vi "Hardware - Buffered Counter Time.vi"(7 "Counter Time Function (Read Timer)":T1=enum."Read Timer", 8 "error in (no error)":errorcluster, 11 "Counter Task In":refnum<k21>) -> (0 "error out":errorcluster, 3 "Timer Value (ms)":dbl caption="Time Value (ms)" format="%#.6g")   [LabVIEW 2010, in "Core SubVIs.lvlib"]
uses:
  Core SubVIs.lvlib
  Controls/TYPE - Count Time Method.ctl
  <vilib>/DAQmx/read.llb/DAQmx Read (Counter 1D U32 1Chan NSamp).vi
  <vilib>/daqmx/miscellaneous.llb/DAQmx Fill In Error Info.vi
  Program Files/National Instruments/LabVIEW 2010/resource/objmgr/daqmx.rc
panel:
  in  "Timebase Rate (10 MHz Default)":dbl=10000000.0 format="%#_6p"
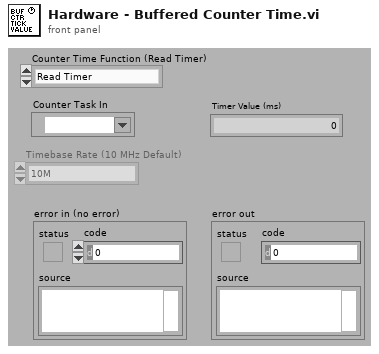
[diagram p1: front panel]
types:
  T1 = typedef "Core SubVIs.lvlib/TYPE - Count Time Method.ctl" = enum16{"Start Timer Task", "Read Timer", "Reset Timer", "Clear Timer Task"}
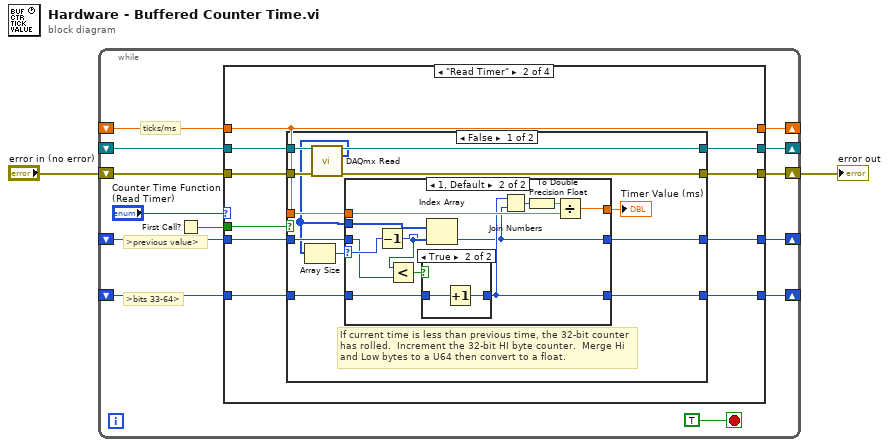
[diagram p0: block diagram]
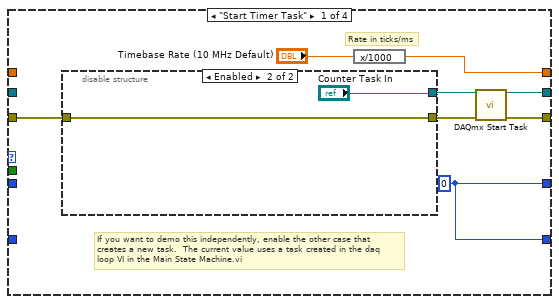
[diagram p2: hidden frame]
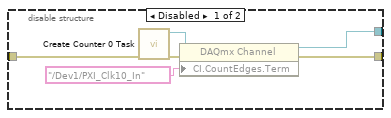
[diagram p3: hidden frame]
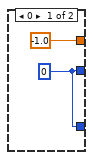
[diagram p4: hidden frame]
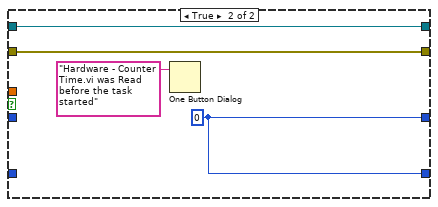
[diagram p6: hidden frame]
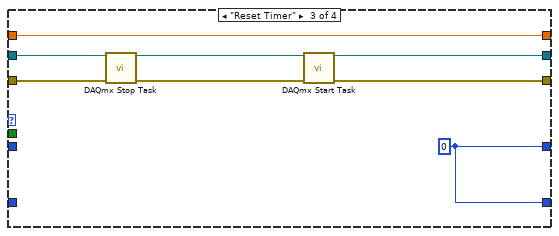
[diagram p7: hidden frame]
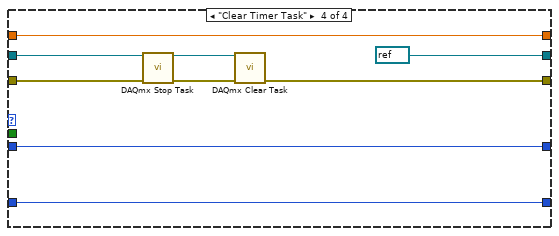
[diagram p8: hidden frame]
diagram:
  n1 = while {
    shift-right: [w12] -> _
    shift-left: _ -> [w15]
    shift-right: [w11] -> w1
    shift-left: "error in (no error)" -> [w14]
    shift-right: [w9] -> _
    shift-left: _ -> [w8]
    shift-right: [w5] -> _
    shift-left: _ -> [w6]
    shift-right: [w3] -> _
    shift-left: _ -> [w4]
    stop <- TRUE stop-if-true
    # ">bits 33-64>"
    # ">previous value>"
    # "ticks/ms"
    n2 = First Call?() -> (First Call?: T/F=w7:bool)
    n3 = case shown="\"Read Timer\"" "Counter Time Function (Read Timer)" {
      tunnel: w15 -> [_ w41 w82 w89]
      tunnel: w14 -> [w20 w40 w81 w88]
      tunnel: [w17 w39 w78 refnum<k21> refnum ("task out")] -> w12
      tunnel: [w18 w38 w77 w87] -> w11
      tunnel: [w22 w32 w76 w85] -> w9
      tunnel: w8 -> [_ w32 w76 w85]
      tunnel: w7 -> [_ w37 _ _]
      tunnel: w6 -> [_ w36 _ w84]
      tunnel: [w21 w35 w75 w84] -> w5
      tunnel: w4 -> [_ w34 _ w83]
      tunnel: [w21 w33 w75 w83] -> w3
      frame "Start Timer Task" {
        w21 = u32 0 ("data")
        # "If you want to demo this independently, enable the other case that\ncreates a new task.  The current value uses a task created in the daq\nloop VI in the Main State Machine.vi"
        # "Rate in ticks/ms"
        n4 = disable-structure shown="Enabled" {
          disable-tunnel: [w24 "Counter Task In"] -> w16
          disable-tunnel: [w25 w30] -> w19
          disable-tunnel: w20 -> [w26 w30]
          frame Disabled {
            n5 = call "Create Counter 0 Task.vi"("error in"=w26) -> ("error out"=w27:errorcluster, "task out"=w28:refnum<k21>)  [unwired: 9 in]
            n6 = property class="DAQmx Channel"(reference=w28, error in=w27, "CI.CountEdges.Term"=tag "/Dev1/PXI_Clk10_In") -> (reference out=w24:refnum<k21>, error out=w25:errorcluster)
          }
          frame Enabled {
          }
        }
        n7 = expression code="x/1000"("Timebase Rate (10 MHz Default)") -> (w22:dbl)
        n8 = call <vilib>:"DAQmx Start Task.vi"("task/channels in"=w16, "error in"=w19) -> ("task out"=w17:refnum<k21>, "error out"=w18:errorcluster)  [unwired: 12 out]
      }
      frame "Read Timer" {
        n9 = case shown="False" w37 {
          tunnel: w41 -> [w48 w74]
          tunnel: w40 -> [w47 w73]
          tunnel: [w46 w74] -> w39
          tunnel: [w45 w73] -> w38
          tunnel: w36 -> [w52 _]
          tunnel: [w42 w71] -> w35
          tunnel: w34 -> [w51 _]
          tunnel: [w50 w71] -> w33
          tunnel: w32 -> [w53 _]
          frame False {
            # "If current time is less than previous time, the 32-bit counter has rolled.  Increment the 32-bit HI byte counter.  Merge Hi and Low bytes to a U64 then convert to a float."
            n10 = call-poly <vilib>:"DAQmx Read.vi"("task/channels in"=w48, "error in"=w47) -> ("task out"=w46:refnum<k21>, "data"=w43:u32[], "error out"=w45:errorcluster)  [unwired: 1 in, 10 out]
            n11 = Array Size(array=w43) -> (size(s)=w44:i32)
            n12 = case shown="1, Default" w44 {
              selector: w44 -> [_ w57]
              tunnel: w53 -> [_ w67]
              tunnel: w52 -> [_ w56]
              tunnel: w51 -> [_ w65]
              tunnel: [w55 w64] -> w50
              tunnel: [-1.0 w62] -> w49
              tunnel: w43 -> [_ w60]
              tunnel: [w55 w59] -> w42
              frame 0 {
                w55 = u32 0 ("Numeric")
              }
              frame 1, Default {
                n13 = Decrement(x=w57) -> (x-1=w58:i32)
                n14 = Index Array(array=w60, index=w58) -> (element=w59:u32)
                n15 = Less?(x=w59, y=w56) -> (x < y?=w66:bool)
                n16 = case shown="True" w66 {
                  tunnel: w65 -> [w68 w70]
                  tunnel: [w68 w69] -> w64
                  frame False {
                  }
                  frame True {
                    n17 = Increment(x=w70) -> (x+1=w69:u32)
                  }
                }
                n18 = Join Numbers(hi=w64, lo=w59) -> ((hi.lo)=w63:u64)
                n19 = To Double Precision Float(number=w63) -> (double precision float=w61:dbl)
                n20 = Divide(x=w61, y=w67) -> (x/y=w62:dbl)
              }
            }
            "Timer Value (ms)" <- w49
          }
          frame True {
            w71 = u32 0 ("data")
            n21 = One Button Dialog(message="Hardware - Counter Time.vi was Read before the task started") -> ()  [unwired: 2 out]
          }
        }
      }
      frame "Reset Timer" {
        w75 = u32 0 ("data")
        n22 = call <vilib>:"DAQmx Stop Task.vi"("task/channels in"=w82, "error in"=w81) -> ("task out"=w80:refnum<k21>, "error out"=w79:errorcluster)  [unwired: 12 out]
        n23 = call <vilib>:"DAQmx Start Task.vi"("task/channels in"=w80, "error in"=w79) -> ("task out"=w78:refnum<k21>, "error out"=w77:errorcluster)  [unwired: 12 out]
      }
      frame "Clear Timer Task" {
        n24 = call <vilib>:"DAQmx Stop Task.vi"("task/channels in"=w89, "error in"=w88) -> ("task out"=w90:refnum<k21>, "error out"=w91:errorcluster)  [unwired: 12 out]
        n25 = call <vilib>:"DAQmx Clear Task.vi"("task in"=w90, "error in"=w91) -> ("error out"=w87:errorcluster)  [unwired: 13 out]
      }
    }
  }
  "error out" <- w1
